vi "ControlsToCluster.vi"(10 "Path (px)":cluster{dbl, dbl}[](array[cluster]), 11 "Path (in)":cluster{dbl, dbl}[](array[cluster])) -> (3 "PathFileData":T1={"RobotNeeded"={"Path"=[], "MaxVel"=0.0, "MaxAccel"=0.0, "Backwards?"=FALSE, "PointSpacing"=0.0, "LookaheadDist"=0.0, "Speed/Curve"=1.8, "SlowDistanceAtEnd"=12.0, "SlowSpeed"=15.0, "MaxDeAccel"=0.0}, "Meta"={"Path (px)"=[], "RobotWidth"=0.0, "RobotLength"=0.0, "CenterOfRotYOffset"=0.0, "Roundedness"=0.0, "StartingPositionPreset"=0, "PathName"=""}} {"RobotNeeded"."SlowSpeed" format="%#_13g"; "RobotNeeded"."SlowDistanceAtEnd" format="%#_13g"; "RobotNeeded"."Speed/Curve" format="%#_13g"})   [LabVIEW 2020]
uses:
  Dawgma Programming Library/Controls/PurePursuit/PathFileData.ctl
  Dawgma Programming Library/Controls/PurePursuit/RobotNeededPathData.ctl
  Robot Project/Configuration/Constants.vi
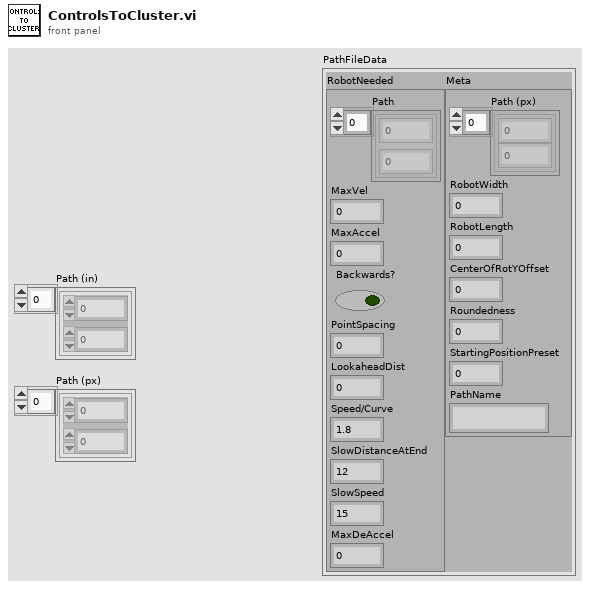
[diagram p1: front panel]
types:
  T1 = typedef "PathFileData.ctl" = cluster{"RobotNeeded":T2, "Meta":cluster{"Path (px)":cluster{i32, i32}[], "RobotWidth":dbl, "RobotLength":dbl, "CenterOfRotYOffset":dbl, "Roundedness":dbl, "StartingPositionPreset":u32, "PathName":string}}
  T2 = typedef "RobotNeededPathData.ctl" = cluster{"Path":cluster{dbl, dbl}[], "MaxVel":dbl, "MaxAccel":dbl, "Backwards?":bool, "PointSpacing":dbl, "LookaheadDist":dbl, "Speed/Curve":dbl, "SlowDistanceAtEnd":dbl, "SlowSpeed":dbl, "MaxDeAccel":dbl}
  T3 = cluster{"Path (px)":cluster{i32, i32}[], "RobotWidth":dbl, "RobotLength":dbl, "CenterOfRotYOffset":dbl, "Roundedness":dbl, "StartingPositionPreset":u32, "PathName":string}
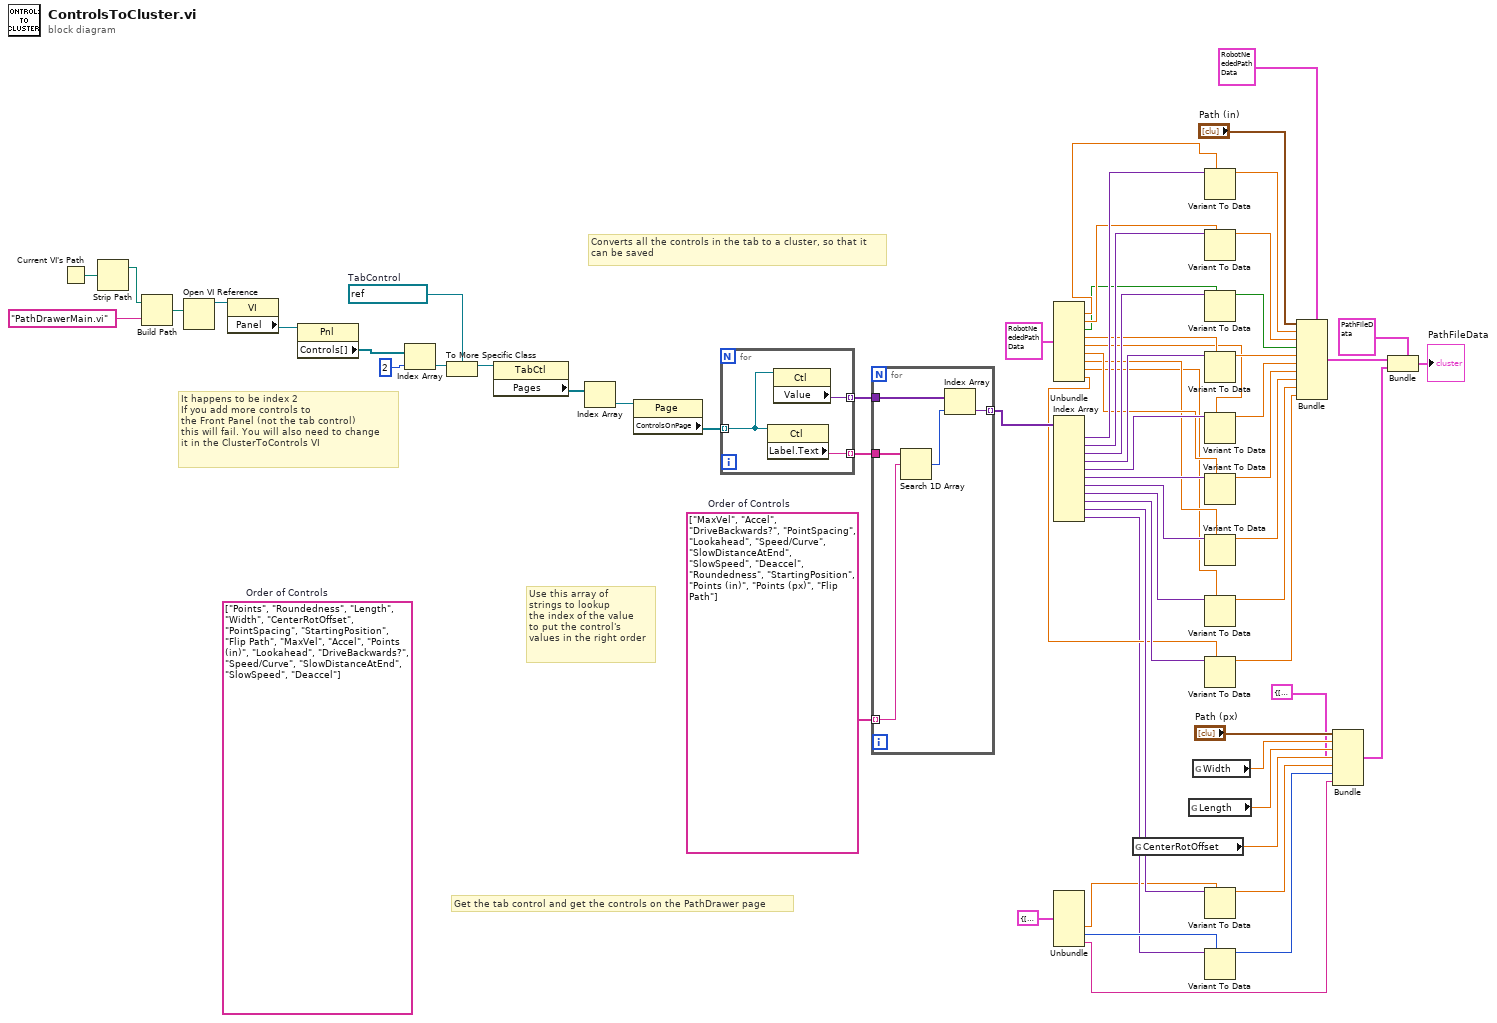
[diagram p0: block diagram]
diagram:
  w42 = string[] ["MaxVel", "Accel", "DriveBackwards?", "PointSpacing", "Lookahead", "Speed/Curve", "SlowDistanceAtEnd", "SlowSpeed", "Deaccel", "Roundedness", "StartingPosition", "Points (in)", "Points (px)", "Flip Path"]  # Order of Controls
  (unwired) string[] ["Points", "Roundedness", "Length", "Width", "CenterRotOffset", "PointSpacing", "StartingPosition", "Flip Path", "MaxVel", "Accel", "Points (in)", "Lookahead", "DriveBackwards?", "Speed/Curve", "SlowDistanceAtEnd", "SlowSpeed", "Deaccel"]  # Order of Controls
  w64 = refnum<vi> refnum  # TabControl
  # "Converts all the controls in the tab to a cluster, so that it\ncan be saved"
  # "Use this array of\nstrings to lookup\nthe index of the value\nto put the control's\nvalues in the right order"
  # "It happens to be index 2\nIf you add more controls to\nthe Front Panel (not the tab control)\nthis will fail. You will also need to change\nit in the ClusterToControls VI"
  # "Get the tab control and get the controls on the PathDrawer page"
  n1 = Current VI's Path() -> (path=w16:path)
  n2 = Strip Path(path=w16) -> (stripped path=w15:path)  [unwired: 1 out]
  n3 = Build Path(base path=w15, name or relative path="PathDrawerMain.vi") -> (appended path=w13:path)
  n4 = Open VI Reference(vi path=w13) -> (vi reference=w12:refnum<vi>)  [unwired: 5 in, 1 out]
  n5 = property class="VI"(reference=w12) -> ("Panel"=w17:refnum<vi>)  [unwired: 1 in, 2 out]
  n6 = property class="Pnl"(reference=w17) -> ("Controls[]"=w11:refnum<vi>[])  [unwired: 1 in, 2 out]
  n7 = Index Array(array=w11, index=2) -> (element=w63:refnum<vi>)
  n8 = To More Specific Class(target class=w64, reference=w63) -> (specific class reference=w62:refnum<vi>)  [unwired: 1 in, 1 out]
  n9 = property class="TabCtl"(reference=w62) -> ("Pages"=w61:refnum<vi>[])  [unwired: 1 in, 2 out]
  n10 = Index Array(array=w61) -> (element=w60:refnum<vi>)  [unwired: 1 in]
  n11 = property class="Page"(reference=w60) -> ("ControlsOnPage"=w59:refnum<vi>[])  [unwired: 1 in, 2 out]
  n12 = for {
    tunnel: w59 -> [w67] mode=indexing
    tunnel: [w68] -> w43 mode=indexing
    tunnel: [w66] -> w44 mode=indexing
    n13 = property class="Ctl"(reference=w67) -> ("Label.Text"=w68:string)  [unwired: 1 in, 2 out]
    n14 = property class="Ctl"(reference=w67) -> ("Value"=w66:variant)  [unwired: 1 in, 2 out]
  }
  n15 = for {
    tunnel: [w69] -> w45 mode=indexing
    tunnel: w44 -> [w71]
    tunnel: w43 -> [w73]
    tunnel: w42 -> [w72] mode=indexing
    n16 = Search 1D Array(1D array=w73, element=w72) -> (index of element=w70:i32)  [unwired: 1 in]
    n17 = Index Array(array=w71, index=w70) -> (element=w69:variant)
  }
  n18 = Unbundle(T2 {"Path"=[], "MaxVel"=0.0, "MaxAccel"=0.0, "Backwards?"=FALSE, "PointSpacing"=0.0, "LookaheadDist"=0.0, "Speed/Curve"=1.8, "SlowDistanceAtEnd"=12.0, "SlowSpeed"=15.0, "MaxDeAccel"=0.0} ("RobotNeededPathData")) -> ("MaxVel"=w41:dbl, "MaxAccel"=w39:dbl, "Backwards?"=w36:bool, "PointSpacing"=w35:dbl, "LookaheadDist"=w32:dbl, "Speed/Curve"=w31:dbl, "SlowDistanceAtEnd"=w29:dbl, "SlowSpeed"=w26:dbl, "MaxDeAccel"=w25:dbl)  [unwired: 1 out]
  n19 = Index Array(array=w45) -> (element #1=w58:variant, element #2=w57:variant, element #3=w56:variant, element #4=w55:variant, element #5=w54:variant, element #6=w53:variant, element #7=w52:variant, element #8=w51:variant, element #9=w50:variant, element #10=w49:variant, element #11=w10:variant)  [unwired: 11 in]
  n20 = Unbundle(T3 {"Path (px)"=[], "RobotWidth"=0.0, "RobotLength"=0.0, "CenterOfRotYOffset"=0.0, "Roundedness"=0.0, "StartingPositionPreset"=0, "PathName"=""} ("Meta")) -> ("Roundedness"=w7:dbl, "StartingPositionPreset"=w20:u32, "PathName"=w3:string)  [unwired: 4 out]
  n21 = global read "Constants.vi" "CenterRotOffset"() -> (w8:dbl)
  n22 = global read "Constants.vi" "Length"() -> (w9:dbl)
  n23 = global read "Constants.vi" "Width"() -> (w5:dbl)
  n24 = Variant To Data(type=w41, Variant=w58) -> (data=w40:dbl)  [unwired: 1 in, 1 out]
  n25 = Variant To Data(type=w39, Variant=w57) -> (data=w38:dbl)  [unwired: 1 in, 1 out]
  n26 = Variant To Data(type=w36, Variant=w56) -> (data=w37:bool)  [unwired: 1 in, 1 out]
  n27 = Variant To Data(type=w35, Variant=w55) -> (data=w34:dbl)  [unwired: 1 in, 1 out]
  n28 = Variant To Data(type=w32, Variant=w54) -> (data=w33:dbl)  [unwired: 1 in, 1 out]
  n29 = Variant To Data(type=w31, Variant=w53) -> (data=w30:dbl)  [unwired: 1 in, 1 out]
  n30 = Variant To Data(type=w29, Variant=w52) -> (data=w28:dbl)  [unwired: 1 in, 1 out]
  n31 = Variant To Data(type=w26, Variant=w51) -> (data=w27:dbl)  [unwired: 1 in, 1 out]
  n32 = Variant To Data(type=w25, Variant=w50) -> (data=w24:dbl)  [unwired: 1 in, 1 out]
  n33 = Variant To Data(type=w7, Variant=w49) -> (data=w6:dbl)  [unwired: 1 in, 1 out]
  n34 = Variant To Data(type=w20, Variant=w10) -> (data=w19:u32)  [unwired: 1 in, 1 out]
  n35 = Bundle(cluster=T2 {"Path"=[], "MaxVel"=0.0, "MaxAccel"=0.0, "Backwards?"=FALSE, "PointSpacing"=0.0, "LookaheadDist"=0.0, "Speed/Curve"=1.8, "SlowDistanceAtEnd"=12.0, "SlowSpeed"=15.0, "MaxDeAccel"=0.0} ("RobotNeededPathData"), "Path"="Path (in)", "MaxVel"=w40, "MaxAccel"=w38, "Backwards?"=w37, "PointSpacing"=w34, "LookaheadDist"=w33, "Speed/Curve"=w30, "SlowDistanceAtEnd"=w28, "SlowSpeed"=w27, "MaxDeAccel"=w24) -> (w18:T2)
  n36 = Bundle(cluster=T3 {"Path (px)"=[], "RobotWidth"=0.0, "RobotLength"=0.0, "CenterOfRotYOffset"=0.0, "Roundedness"=0.0, "StartingPositionPreset"=0, "PathName"=""} ("Meta"), "Path (px)"="Path (px)", "RobotWidth"=w5, "RobotLength"=w9, "CenterOfRotYOffset"=w8, "Roundedness"=w6, "StartingPositionPreset"=w19, "PathName"=w3) -> (w2:T3)
  n37 = Bundle(cluster=T1 {"RobotNeeded"={"Path"=[], "MaxVel"=0.0, "MaxAccel"=0.0, "Backwards?"=FALSE, "PointSpacing"=0.0, "LookaheadDist"=0.0, "Speed/Curve"=1.8, "SlowDistanceAtEnd"=12.0, "SlowSpeed"=15.0, "MaxDeAccel"=0.0}, "Meta"={"Path (px)"=[], "RobotWidth"=0.0, "RobotLength"=0.0, "CenterOfRotYOffset"=0.0, "Roundedness"=0.0, "StartingPositionPreset"=0, "PathName"=""}} ("Data"), "RobotNeeded"=w18, "Meta"=w2) -> (→"PathFileData":T1)
